vi "get_relays.vi"(8 "error in (no error)":errorcluster, 9 "card address":u8=1, 11 "VISA Refnum in":refnum<visa-resource-name>) -> (0 "error out":errorcluster, 1 "return string":string, 2 "boolian array out":bool[](array[boolean]), 3 "VISA Refnum out":refnum<visa-resource-name>)   [LabVIEW 2018]
doc: "Command 2 is issued.\nGet the status all 8 relays of the selected card (card number)."
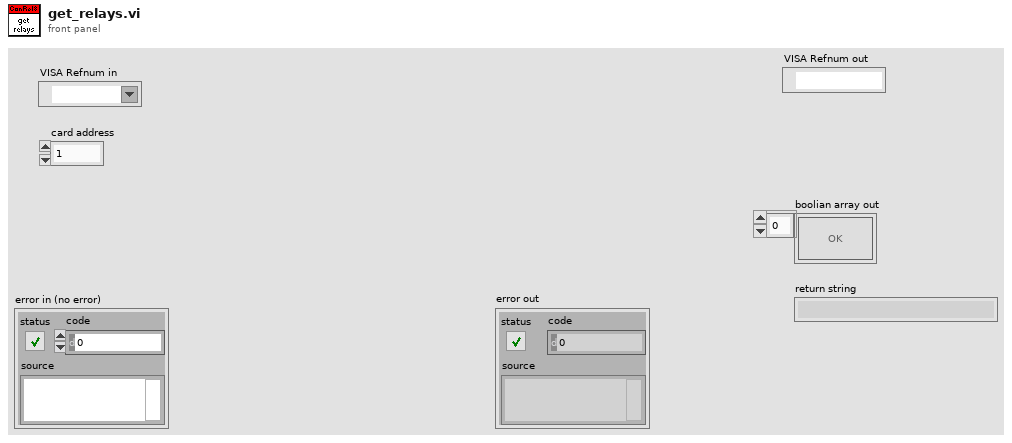
[diagram p1: front panel]
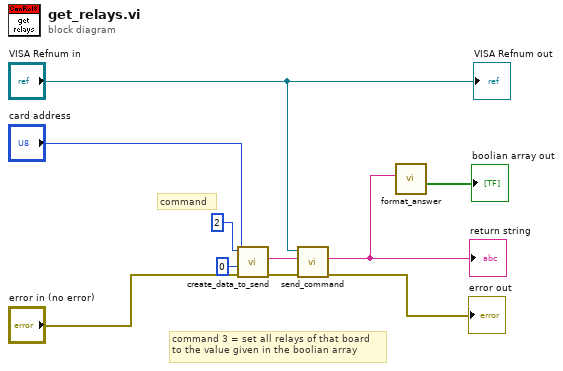
[diagram p0: block diagram]
diagram:
  # "command 3 = set all relays of that board\nto the value given in the boolian array"
  # "command"
  n1 = call "create_data_to_send.vi"("error in (no error)"="error in (no error)", "data"=u8 0, "address"="card address", "command"=u8 2) -> ("error out"=w8:errorcluster, "send string"=w10:string)  [unwired: 4 in, 2 out]
  n2 = call "send_command.vi"("error in (no error)"=w8, "command"=w10, "VISA Refnum in"="VISA Refnum in") -> ("error out"=→"error out":errorcluster, "return string"=w2:string)  [unwired: 5 in, 2 out]
  "return string" <- w2
  n3 = call "format_answer.vi"("answer string"=w2) -> ("switches"=→"boolian array out":bool[])  [unwired: 6 in, 4 out]
  "VISA Refnum out" <- "VISA Refnum in"
